vi "_CmdExe._Dummy VI with time delay.vi"(11 "Timeout":dbl=5.0) -> ()   [LabVIEW 2024]
uses:
  <vilib>/KATE/Time/Time Utils.lvlib
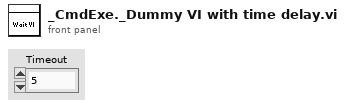
[diagram p1: front panel]
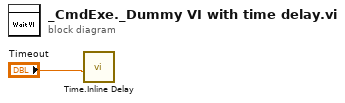
[diagram p0: block diagram]
diagram:
  n1 = call <vilib>:"Time.Inline Delay.vi"("Wait(secs)"="Timeout") -> ()  [unwired: 9 in, 2 out]
